vi "Create Trigger Model Buffer Clear Block.vi"(8 "error in (no error)":errorcluster, 9 "Buffer Name (defbuffer1)":string, 10 "Block Number (1)":i32 min=1 format="%#.6g", 11 "VISA resource name":refnum<visa-resource-name>) -> (0 "error out":errorcluster, 3 "VISA resource name out":refnum<visa-resource-name>)   [LabVIEW 2009, in "Keithley DMM7510.lvlib"]
doc: "This VI defines a trigger model block that clears the reading buffer."
uses:
  Keithley DMM7510.lvlib
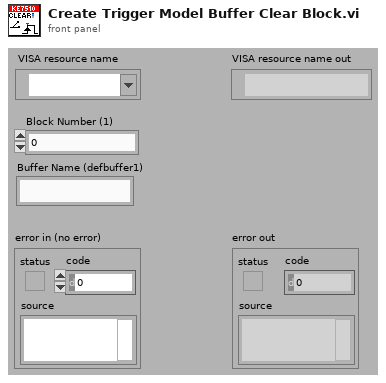
[diagram p1: front panel]
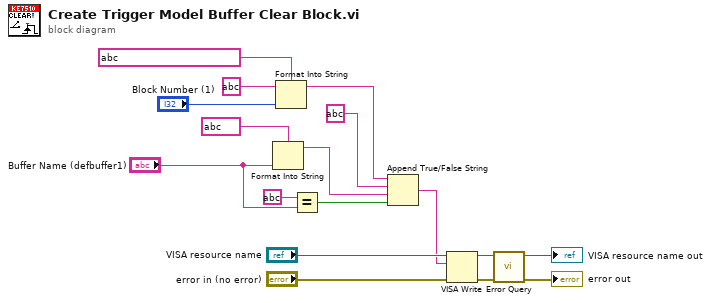
[diagram p0: block diagram]
diagram:
  n1 = Format Into String(format string=string ?, "Buffer Name (defbuffer1)") -> (resulting string=w5:string)  [unwired: 2 in, 1 out]
  n2 = Format Into String(format string=string ?, initial string=string ?, "Block Number (1)") -> (resulting string=w3:string)  [unwired: 1 in, 1 out]
  n3 = Equal?(x=string ? ("y"), y="Buffer Name (defbuffer1)") -> (x = y?=w4:bool)
  n4 = Append True/False String(1:w4, 2:w5, 3:string ? ("true string"), 4:w3) -> (0:w6:string)
  n5 = VISA Write(VISA resource name="VISA resource name", write buffer=w6, error in (no error)="error in (no error)") -> (VISA resource name out=w13:refnum<visa-resource-name>, error out=w12:errorcluster)  [unwired: 1 out]
  n6 = call "Error Query.vi"("error in (no error)"=w12, "VISA resource name"=w13) -> ("error out"=→"error out":errorcluster, "VISA resource name out"=→"VISA resource name out":refnum<visa-resource-name>)  [unwired: 8 out]
